vi "Control Drivetrain.vi"(11 "Loop Time (ms)":u32) -> ()   [LabVIEW 2017]
uses:
  <vilib>/Rock Robotics/WPI/DriverStation/WPI_DriverStationRobotMode2.ctl
  Globals/Robot Global Data.vi
  <vilib>/Rock Robotics/WPI/Utilities/WPI_GetSetVariantRefNum.vi
  <vilib>/Rock Robotics/WPI/RobotDrive/WPI_RobotDriveArcadeDrive_Standard(NoSaturation).vi
  <vilib>/Rock Robotics/Network Tables/NT Write Numeric Array.vi
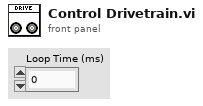
[diagram p1: front panel]
types:
  T1 = typedef "WPI_DriverStationRobotMode2.ctl" = enum16{"Autonomous Disabled", "Autonomous Enabled", "Teleop Disabled", "Teleop Enabled", "Disconnected", "Finish", "Test Disabled", "Test Enabled", "Emergency Stopped"}
  T2 = typedef "WPI_RobotDriveDevRef.ctl" = cluster{"DevStatus":errorcluster, "Motors[]":T3[], "Square Inputs":bool, "Max Output":dbl}
  T3 = typedef "WPI_MotorControlDeviceRef.ctl" = cluster{"DeviceStatus":errorcluster, "Type":T4, "PWM":cluster{"PWM Channel":T5, "DeadBand":T6}, "CAN":cluster{"Device Number":u8, "SetOutput VI Ref":variant, "GetOutput VI Ref":variant, "Enable VI Ref":variant, "Disable VI Ref":variant, "Data":variant}, "Invert":bool, "DIO PWM":cluster{"PWM \"Enable\" Channel":T5, "DIOChannel":T7, "PWM Rate":dbl}}
  T4 = typedef "WPI_MotorControlType.ctl" = enum16{"PWM", "CAN", "DIO PWM"}
  T5 = typedef "FPGA_DIOPWMChannel.ctl" = enum8{"PWM 0", "PWM 1", "PWM 2", "PWM 3", "PWM 4", "PWM 5", "PWM 6", "PWM 7", "PWM 8", "PWM 9", "PWM MXP 0", "PWM MXP 1", "PWM MXP 2", "PWM MXP 3", "PWM MXP 4", "PWM MXP 5", "PWM MXP 6", "PWM MXP 7", "PWM MXP 8", "PWM MXP 9", "Invalid"}
  T6 = typedef "WPI_PWMDeadband.ctl" = cluster{"Name":string, "maxPositivePwm":i32, "minPositivePwm":i32, "centerPwm":i32, "maxNegativePwm":i32, "minNegativePwm":i32, "angularRange":u16}
  T7 = typedef "FPGA_DIOChannel.ctl" = enum8{"DIO 0", "DIO 1", "DIO 2", "DIO 3", "DIO 4", "DIO 5", "DIO 6", "DIO 7", "DIO 8", "DIO 9", "DIO MXP 0", "DIO MXP 1", "DIO MXP 2", "DIO MXP 3", "DIO MXP 4", "DIO MXP 5", "DIO MXP 6", "DIO MXP 7", "DIO MXP 8", "DIO MXP 9", "DIO MXP 10", "DIO MXP 11", "DIO MXP 12", "DIO MXP 13", "DIO MXP 14", "DIO MXP 15", "SPI Port CS1", "SPI Port CS2", "SPI Port CS3", "SPI Port MISO", "SPI Port MOSI", "Invalid"}
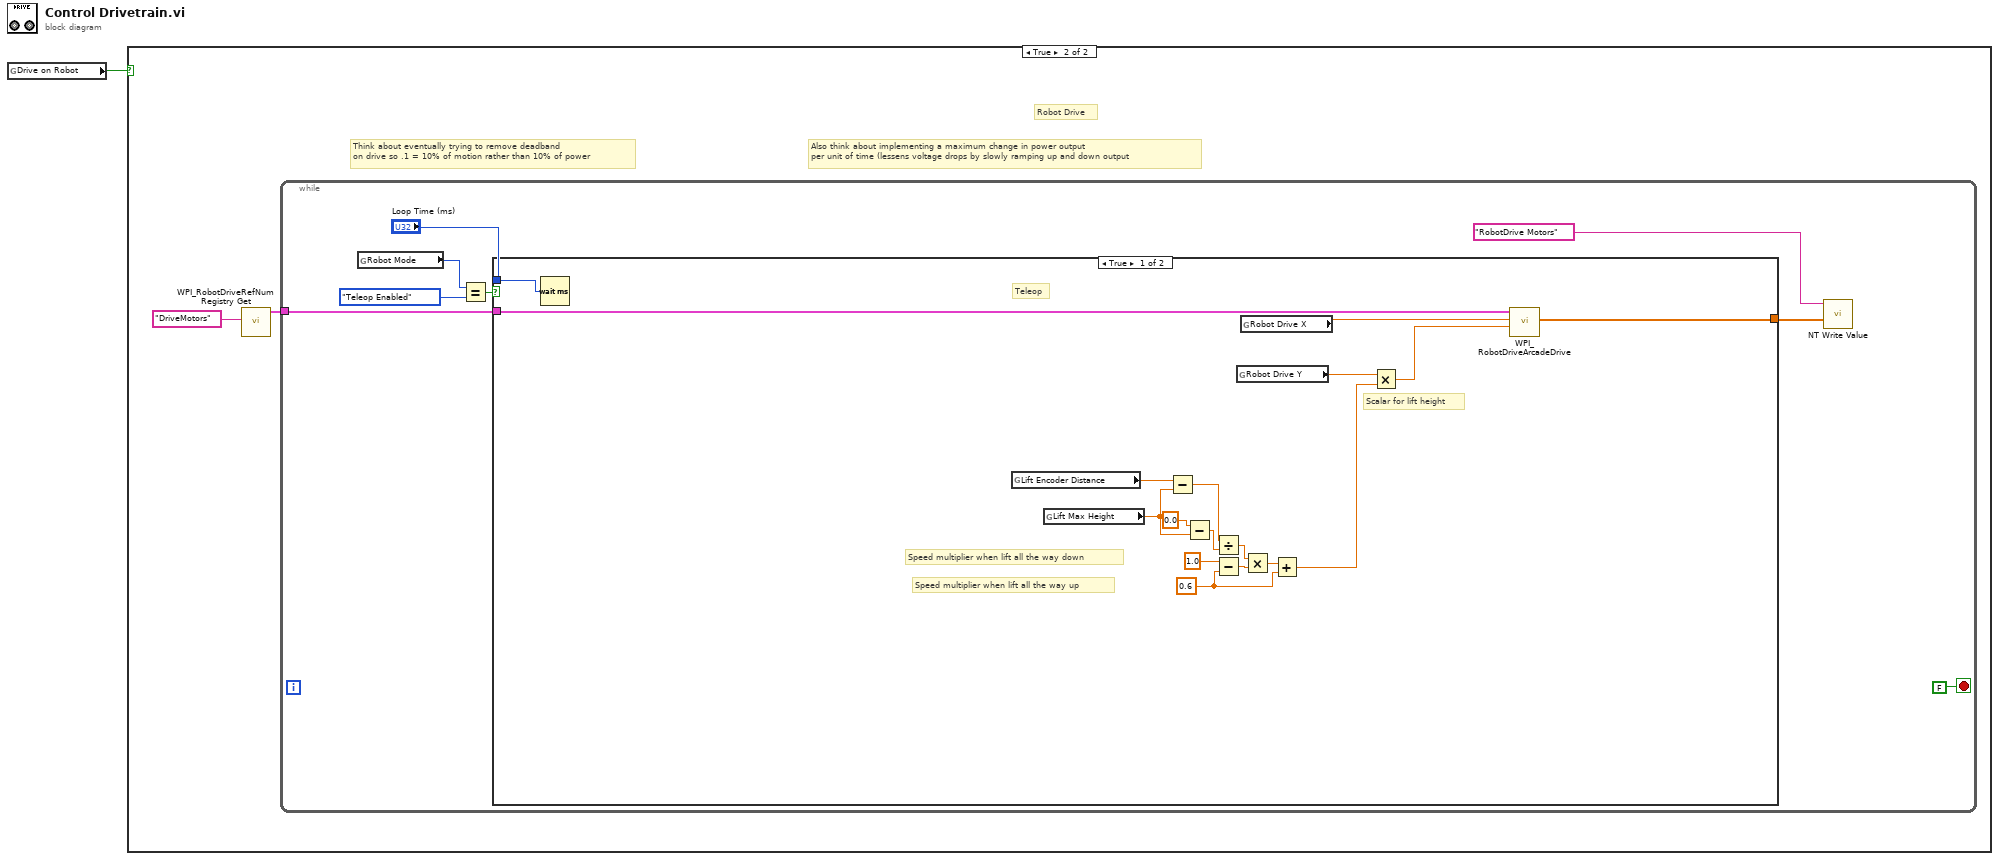
[diagram p0: block diagram]
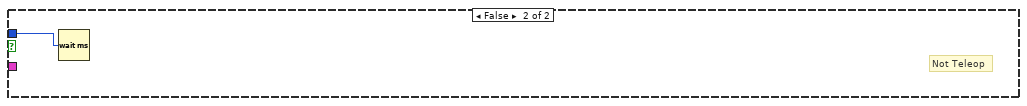
[diagram p3: hidden frame]
diagram:
  n1 = global read "Robot Global Data.vi" "Drive on Robot"() -> (w1:bool)
  n2 = case shown="True" w1 {
    frame False {
    }
    frame True {
      # "Robot Drive"
      # "Also think about implementing a maximum change in power output\nper unit of time (lessens voltage drops by slowly ramping up and down output"
      # "Think about eventually trying to remove deadband\non drive so .1 = 10% of motion rather than 10% of power"
      n3 = call <vilib>:"WPI_RobotDriveRefNum Registry Get.vi"("refnum name"="DriveMotors") -> ("RobotDriveDevRef"=w2:T2)  [unwired: 9 in, 1 out]
      n4 = while {
        tunnel: w2 -> [w8]
        stop <- FALSE stop-if-true
        n5 = global read "Robot Global Data.vi" "Robot Mode"() -> (w10:T1)
        n6 = Equal?(x=w10, y=WPI_DriverStationRobotMode2."Teleop Enabled") -> (x = y?=w11:bool)
        n7 = case shown="True" w11 {
          tunnel: w8 -> [w28 _]
          tunnel: "Loop Time (ms)" -> [w27 w29]
          tunnel: [w26 _] -> w6
          frame True {
            w15 = 0.6
            # "Scalar for lift height"
            # "Speed multiplier when lift all the way up"
            # "Speed multiplier when lift all the way down"
            # "Teleop"
            n8 = Wait (ms)(milliseconds to wait=w27) -> ()  [unwired: 1 out]
            n9 = global read "Robot Global Data.vi" "Lift Encoder Distance"() -> (w24:dbl)
            n10 = global read "Robot Global Data.vi" "Lift Max Height"() -> (w22:dbl)
            n11 = Subtract(x=w24, y=w22) -> (x-y=w21:dbl)
            n12 = Subtract(x=0.0, y=w22) -> (x-y=w20:dbl)
            n13 = Divide(x=w21, y=w20) -> (x/y=w19:dbl)
            n14 = Subtract(x=1.0, y=w15) -> (x-y=w17:dbl)
            n15 = global read "Robot Global Data.vi" "Robot Drive Y"() -> (w13:dbl)
            n16 = global read "Robot Global Data.vi" "Robot Drive X"() -> (w25:dbl)
            n17 = Multiply(x=w19, y=w17) -> (x*y=w16:dbl)
            n18 = Add(x=w16, y=w15) -> (x+y=w12:dbl)
            n19 = Multiply(x=w13, y=w12) -> (x*y=w14:dbl)
            n20 = call-poly <vilib>:"WPI_RobotDriveArcadeDrive.vi"("Y axis value"=w14, "X axis value"=w25, "RobotDriveDevRef"=w28) -> ("Motor Values"=w26:dbl[])  [unwired: 6 in, 2 out]
          }
          frame False {
            # "Not Teleop"
            n21 = Wait (ms)(milliseconds to wait=w29) -> ()  [unwired: 1 out]
          }
        }
        n22 = call-poly <vilib>:"NT Write Value.vi"("Numeric Array"=w6, "Name"="RobotDrive Motors") -> ()  [unwired: 9 in, 1 out]
      }
    }
  }
